vi "AlliGator Get Single Saved Dataset Path.vi"(8 "error in (no error)":errorcluster, 10 "Original Dataset Name without Extension":string, 11 "Single Dataset Path":path) -> (0 "error out":errorcluster, 1 "Current Frame in Dataset":i32, 2 "# Frames in Dataset":i32, 3 "Single Dataset Path":path)   [LabVIEW 2021, in "AlliGator Files.lvlib"]
doc: "Builds path for saved HFD5 FLI Dataset file."
uses:
  AlliGator Files.lvlib
  AlliGator Variables List.ctl
  Variant/Variant to Data/Variant to I32.vi
  AlliGator Globals, Variables & Constants.lvlib
  Variant/Variant to Data/Variant to Data.lvlib
panel:
  # "see the AlliGator License on the block diagram (Ctrl+E or Window:Show Block Diagram)"
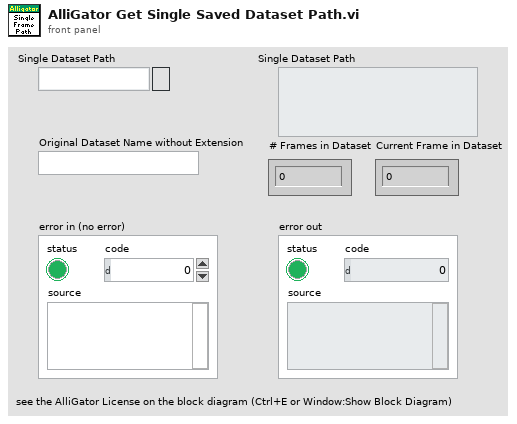
[diagram p1: front panel]
types:
  T1 = typedef "AlliGator Globals, Variables & Constants.lvlib/AlliGator Variables List.ctl" = enum16{"---- GUI ----", "GUI:Initialization Status", "GUI:State Indicators Refnum", "GUI:Original AlliGator Menu Items", "GUI:Current Action Loop State", "GUI:Script in progress", "GUI:Playback", "GUI:Loop Playback", "GUI:Search ROI Used", "GUI:Search ROI", "Decay Graph Max Legend Size", "Intensity Graph Max Legend Size", "Decay Statistics Graph Max Legend Size", "Phasor Graph Max Legend Size", "Phasor Ratio Graph Max Legend Size", "Lifetime Graph Max Legend Size", "---- Files ----", "Files:Export Dataset Frames as Individual Files", "Files:Show Batch Export Help Balloons", "Files:Frames in Dataset", "Files:ptu File Frame Start Indices", "Files:Current Frame in Dataset", "Files:Current Frame Timestamp", "Files:Dataset Loaded", "Files:Dataset Metadata", "Files:Dataset Channel", "Files:Dataset Data Description", "Files:Background Dataset Metadata", "Files:Background Dataset Channel", "Files:Background Dataset Data Description", "Files:Background File Subtraction", "Files:Background File Path", "Files:Background File Pile-up Correction", "Files:Background File Pixel Well Capacity", "Files:Background File Scaling Factor", "Files:Current Dataset Load Settings", "Files:Dataset Path", "Files:ICCD-specific Information", "Files:Macrotime Gate Separation", "------ Python Plugins ------", "Python Plugins:Information", "Python Plugins:Python Session", "Python Plugins:Valid Python Session?", "---- Source Image ----", "Source Image:ROIs", "Source Image:Current ROI", "Source Image:ROI Event Refnum", "X_Source Image Display Range", "X_Source Image Palette Information", "X_Type of Displayed Image", "X_Time Gate Slider", "Source Image:Palette List", "Source Image:Scale", "Source Image:ROI Overlay Color", "Source Image:Overlay to Erase", "Source Image:Is Displayed Image Accumulated", "Source Image:White Light Image Modified", "Source Image:Mask Image Modified", "---- Image Profile Window ----", "Image Profile:Overlay ROI in Source Image", "Image Profile:Window Event Refnum", "Image Profile:IntensityType", "Image Profile:Intensity Average Type", "Image Profile:Intensity-weighted SDV", "Image Profile:Box Profile Type", "Image Profile:Window Open", "Image Profile:Plotted Fit Parameter", "------ Phasor Graph -------", "Phasor Graph:Show Line", "---- Phasor Plot ---", "Phasor Plot:Parameters Changed", "Phasor Plot:FLI Dataset Modified since last Calculation", "Phasor Harmonics Data", "Selected Phasor Harmonics", "Phasor Harmonic Manager Event Refnum", "Phasor Plot:ROIs", "Phasor Plot:Current ROI", "Phasor Plot:ROI Event Refnum", "Phasor Plot:Image Reference Points", "Phasor Plot:Computed", "Phasor Plot:Palette Information", "Phasor Plot:Palette List", "Phasor Plot:Phasor Ratio Palette Information", "Phasor Plot:Phasor Ratio Palette List", "Phasor Plot:Image Scale", "Phasor Plot:Image Overlay to Erase", "Phasor Plot:Image Elements to Update", "Phasor Plot:Current Calculation Parameters", "Phasor Plot:Current Calibration Options", "Phasor Plot:Reset Cumulated Phasor Plot", "Phasor Plot:Reference 1", "Phasor Plot:Lifetime Reference 1", "Phasor Plot:Reference 1 Frequency", "Phasor Plot:Reference 2", "Phasor Plot:Lifetime Reference 2", "Phasor Plot:Reference 2 Frequency", "---- Decay Analysis ----", "Number of Selected Decays to Fit", "LS Fit Results", "LAR Fit Results", "BS Fit Results", "Last Decay Max - Min", "Best Fit Parameters", "Best Fit Parameter Names", "Actual Size X", "Actual Size Y", "Binning X", "Binning Y", "Actual # Gates", "Dataset Number", "Gates to...", "Gates Skipped", "Gates to keep", "Gate Step", "Gate Separation", "Reversed Gates", "Pile-up Correction", "Pixel Well Capacity", "Background Subtracted", "Background Subtraction Method", "Background Definition Range", "Background File (deprecated)", "Number of Dataset Accumulated", "Array of Accumulated Dataset Paths", "Do Averaged Datasets", "Destination File Path", "Process Plot Target", "Use 1/D as Phasor Frequency", "---- Decay Fit Parameter Map -----", "Decay Fit Parameter Map:Palette Information", "Decay Fit Parameter Map:Palette List", "------- Local Decay Window ---------", "Local Decay Graph Window:Event Refnum", "Local Decay Graph Window:Use normalized IRF for convolution", "----- Miscellaneous ----", "Misc:Skippable Dialog Windows Status"}
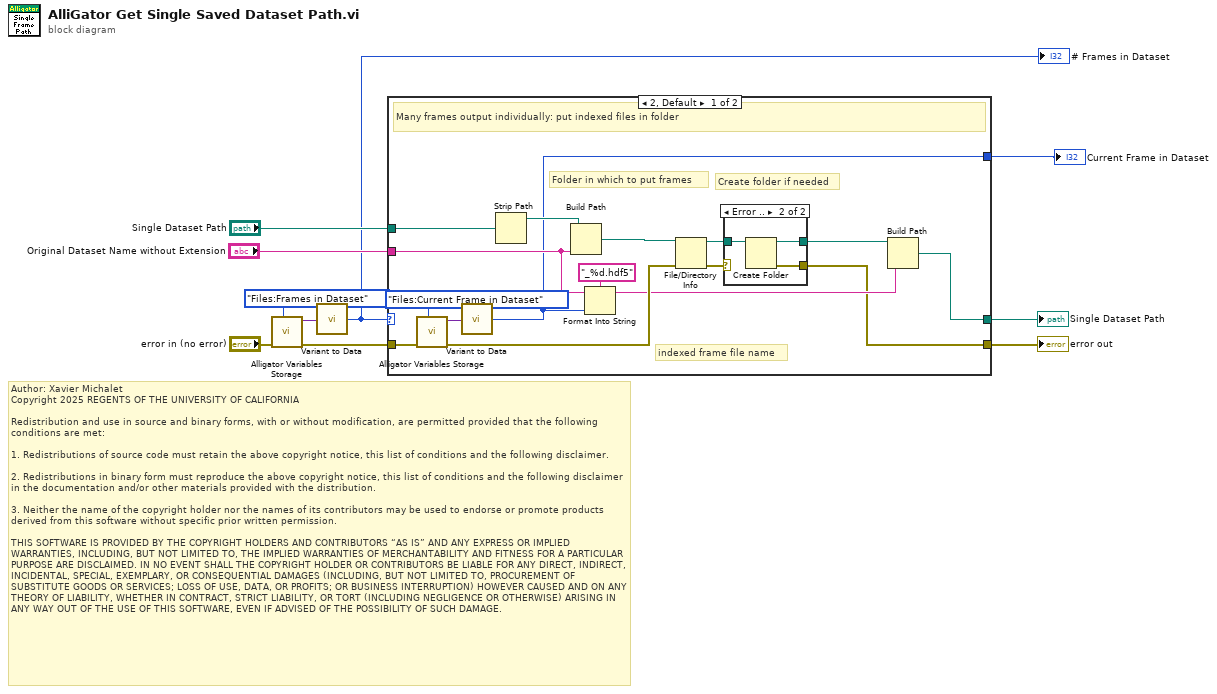
[diagram p0: block diagram]
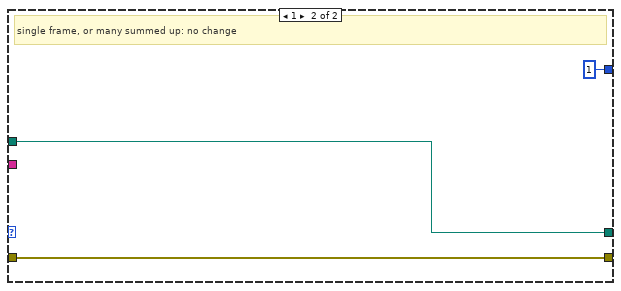
[diagram p3: hidden frame]
diagram:
  # "Author: Xavier Michalet\nCopyright 2025 REGENTS OF THE UNIVERSITY OF CALIFORNIA\n\nRedistribution and use in source and binary forms, with or without modification, are permitted provided that the following conditions are met:\n\n1. Redistributions of source code must retain the above copyright notice, this list of conditions and the following disclaimer.\n\n2. Redistributions in binary form must reproduce the above copyright notice, this list of conditions and the following disclaimer in the documentation and/or other materials provided with the distribution.\n\n3. Neither the name of the copyright holder nor the names of its contributors may be used to endorse or promote products derived from this software without specific prior written permission.\n\nTHIS SOFTWARE IS PROVIDED BY THE COPYRIGHT HOLDERS AND CONTRIBUTORS “AS IS” AND ANY EXPRESS OR IMPLIED WARRANTIES, INCLUDING, BUT NOT LIMITED TO, THE IMPLIED WARRANTIES OF MERCHANTABILITY AND FITNESS FOR A PARTICULAR PURPOSE ARE DISCLAIMED. IN NO EVENT SHALL THE COPYRIGHT HOLDER OR CONTRIBUTORS BE LIABLE FOR ANY DIRECT, INDIRECT, INCIDENTAL, SPECIAL, EXEMPLARY, OR CONSEQUENTIAL DAMAGES (INCLUDING, BUT NOT LIMITED TO, PROCUREMENT OF SUBSTITUTE GOODS OR SERVICES; LOSS OF USE, DATA, OR PROFITS; OR BUSINESS INTERRUPTION) HOWEVER CAUSED AND ON ANY THEORY OF LIABILITY, WHETHER IN CONTRACT, STRICT LIABILITY, OR TORT (INCLUDING NEGLIGENCE OR OTHERWISE) ARISING IN ANY WAY OUT OF THE USE OF THIS SOFTWARE, EVEN IF ADVISED OF THE POSSIBILITY OF SUCH DAMAGE."
  n1 = call "Alligator Variables Storage.vi"("AlliGator Variable"=AlliGator_Variables_List."Files:Frames in Dataset" ("Alligator Variable"), "Error In"="error in (no error)") -> ("Error Out"=w8:errorcluster, "Data out"=w4:variant)  [unwired: 7 in, 1 out]
  n2 = call-poly "Variant to Data.vi"("Variant"=w4) -> ("Value"=w2:i32)  [unwired: 8 in]
  "# Frames in Dataset" <- w2
  n3 = case shown="2, Default" w2 {
    tunnel: "Single Dataset Path" -> [w20 w34]
    tunnel: [w17 w34] -> w6
    tunnel: w8 -> [w25 w33]
    tunnel: [w14 w33] -> w9
    tunnel: "Original Dataset Name without Extension" -> [w21 _]
    tunnel: [w11 1 ("Value")] -> w1
    frame 2, Default {
      # "Create folder if needed"
      # "indexed frame file name"
      # "Folder in which to put frames"
      # "Many frames output individually: put indexed files in folder"
      n4 = call "Alligator Variables Storage.vi"("AlliGator Variable"=AlliGator_Variables_List."Files:Current Frame in Dataset" ("Alligator Variable"), "Error In"=w25) -> ("Error Out"=w23:errorcluster, "Data out"=w26:variant)  [unwired: 7 in, 1 out]
      n5 = call-poly "Variant to Data.vi"("Variant"=w26) -> ("Value"=w11:i32)  [unwired: 8 in]
      n6 = Strip Path(path=w20) -> (stripped path=w15:path)  [unwired: 1 out]
      n7 = Build Path(base path=w15, name or relative path=w21) -> (appended path=w19:path)
      n8 = Format Into String(format string="_%d.hdf5", initial string=w21, w11) -> (resulting string=w18:string)  [unwired: 1 in, 1 out]
      n9 = File/Directory Info(path=w19, error in=w23) -> (path out=w13:path, error out=w16:errorcluster)  [unwired: 5 out]
      n10 = case shown="Error .." w16 {
        selector: w16 -> [w28 _]
        tunnel: [w28 w31] -> w14
        tunnel: w13 -> [w27 w30]
        tunnel: [w27 w29] -> w12
        frame No Error {
        }
        frame Error {
          n11 = Create Folder(path (use dialog)=w30) -> (created path=w29:path, error out=w31:errorcluster)  [unwired: 2 in, 1 out]
        }
      }
      n12 = Build Path(base path=w12, name or relative path=w18) -> (appended path=w17:path)
    }
    frame 1 {
      # "single frame, or many summed up: no change"
    }
  }
  "error out" <- w9
  "Single Dataset Path" <- w6
  "Current Frame in Dataset" <- w1
